vi "Main.vi"(7 "sweep rate, /min":dbl=0.2, 8 "sweep to:":dbl=4.0, 9 "sweep":T8(radio)=enum."2636a_smub") -> ()   [LabVIEW 2021] (continued)
                          n4492 = property on="Offset_super" class="DigNum (strict)"() -> ("Value"=w5886:dbl)  [unwired: 2 in, 2 out]
                          n4493 = property on="Slope_super" class="DigNum (strict)"() -> ("Value"=w5887:dbl)  [unwired: 2 in, 2 out]
                          n4494 = Multiply(x=w5893, y=w5887) -> (x*y=w5892:dbl)
                          n4495 = Add(x=w5892, y=w5886) -> (x+y=w5889:dbl)
                          n4496 = call "setLevel.vi"("VISA resource name 2"=w5888, "Source"=Source."Voltage", "Channel"=Channel."a", "SourceLevel"=w5889) -> ()  [unwired: 1 in, 3 out]
                        }
                      }
                      n4497 = property on="SuperHyper" class="DigNum (strict)"("Value"=w5874) -> ()  [unwired: 2 in, 2 out]
                    }
                  }
                  frame "time_SuperHyper", Default {
                    # "do not sweep, just time"
                  }
                  frame "iPS_SuperHyper" {
                    # "step magnetic field"
                    n4498 = stacked-sequence {
                      tunnel: w5894 -> [_ _ _ _ w5909 _ _ _ w5921 _ w5924 _]
                      frame #0 {
                        n4499 = property on="SuperHyper_Index" class="DigNum (strict)"() -> ("Value"=w5895:dbl)  [unwired: 2 in, 2 out]
                        n4500 = Equal?(x=w5895, y=0.0) -> (x = y?=w5896:bool)
                        n4501 = case shown="True" w5896 {
                          frame False {
                          }
                          frame True {
                            n4502 = property on="iPS _addr_superhyper" class="VISAName"() -> ("Value"=w5900:refnum<visa-resource-name>)  [unwired: 2 in, 2 out]
                            n4503 = property on="Super_FieldRate\n(T/min)" class="DigNum (strict)"() -> ("Value"=w5899:dbl)  [unwired: 2 in, 2 out]
                            n4504 = call "iPSset.vi"("Field Rate, T/min"=w5899, "iPSSetCtrl"=iPSsetCtrl."Set Target Field Rate", "VISA resource name"=w5900) -> ("VISA resource name out"=w5898:refnum<visa-resource-name>)  [unwired: 5 in, 3 out]
                            n4505 = property on="iPS _addr_superhyper" class="VISAName"("Value"=w5898) -> ()  [unwired: 2 in, 2 out]
                          }
                        }
                      }
                      frame #1 {
                        n4506 = Wait (ms)(milliseconds to wait=u32 500) -> ()  [unwired: 1 out]
                      }
                      frame #2 {
                        n4507 = property on="iPS _addr_superhyper" class="VISAName"() -> ("Value"=w5904:refnum<visa-resource-name>)  [unwired: 2 in, 2 out]
                        n4508 = call "iPSset.vi"("iPSSetCtrl"=iPSsetCtrl."Hold", "VISA resource name"=w5904) -> ("VISA resource name out"=w5903:refnum<visa-resource-name>)  [unwired: 6 in, 3 out]
                        n4509 = property on="iPS _addr_superhyper" class="VISAName"("Value"=w5903) -> ()  [unwired: 2 in, 2 out]
                      }
                      frame #3 {
                        n4510 = Wait (ms)(milliseconds to wait=u32 500) -> ()  [unwired: 1 out]
                      }
                      frame #4 {
                        n4511 = property on="iPS _addr_superhyper" class="VISAName"() -> ("Value"=w5908:refnum<visa-resource-name>)  [unwired: 2 in, 2 out]
                        n4512 = call "iPSset.vi"("Target Field, T"=w5909, "iPSSetCtrl"=iPSsetCtrl."Set Target Field", "VISA resource name"=w5908) -> ("VISA resource name out"=w5907:refnum<visa-resource-name>)  [unwired: 5 in, 3 out]
                        n4513 = property on="iPS _addr_superhyper" class="VISAName"("Value"=w5907) -> ()  [unwired: 2 in, 2 out]
                      }
                      frame #5 {
                        n4514 = Wait (ms)(milliseconds to wait=u32 500) -> ()  [unwired: 1 out]
                      }
                      frame #6 {
                        n4515 = property on="iPS _addr_superhyper" class="VISAName"() -> ("Value"=w5912:refnum<visa-resource-name>)  [unwired: 2 in, 2 out]
                        n4516 = call "iPSset.vi"("iPSSetCtrl"=iPSsetCtrl."Hold", "VISA resource name"=w5912) -> ("VISA resource name out"=w5913:refnum<visa-resource-name>)  [unwired: 6 in, 3 out]
                        n4517 = property on="iPS _addr_superhyper" class="VISAName"("Value"=w5913) -> ()  [unwired: 2 in, 2 out]
                      }
                      frame #7 {
                        n4518 = Wait (ms)(milliseconds to wait=u32 500) -> ()  [unwired: 1 out]
                      }
                      frame #8 {
                        n4519 = Equal To 0?(x=w5921) -> (x = 0?=w5920:bool)
                        n4520 = property on="iPS _addr_superhyper" class="VISAName"() -> ("Value"=w5916:refnum<visa-resource-name>)  [unwired: 2 in, 2 out]
                        n4521 = Select(t=iPSsetCtrl."Go to Zero" ("iPSSetCtrl"), s=w5920, f=iPSsetCtrl."Go to Field" ("iPSSetCtrl")) -> (s? t:f=w5917:T16)
                        n4522 = call "iPSset.vi"("iPSSetCtrl"=w5917, "VISA resource name"=w5916) -> ()  [unwired: 6 in, 4 out]
                      }
                      frame #9 {
                        n4523 = Wait (ms)(milliseconds to wait=u32 500) -> ()  [unwired: 1 out]
                      }
                      frame #10 {
                        n4524 = while {
                          tunnel: w5924 -> [w5955]
                          stop <- w5948 stop-if-true
                          n4525 = property on="iPS _addr_superhyper" class="VISAName"() -> ("Value"=w5951:refnum<visa-resource-name>)  [unwired: 2 in, 2 out]
                          n4526 = call "iPSread.vi"("iPSreadCtrl"=iPSreadCtrl."MagnetField", "VISA resource name"=w5951) -> ("number"=w5949:dbl, "VISA resource name out"=w5950:refnum<visa-resource-name>)  [unwired: 6 in, 2 out]
                          n4527 = property on="Tolerance_super" class="DigNum (strict)"() -> ("Value"=w5947:dbl)  [unwired: 2 in, 2 out]
                          n4528 = Wait (ms)(milliseconds to wait=u32 500) -> ()  [unwired: 1 out]
                          n4529 = Subtract(x=w5949, y=w5955) -> (x-y=w5954:dbl)
                          n4530 = property on="iPS _addr_superhyper" class="VISAName"("Value"=w5950) -> ()  [unwired: 2 in, 2 out]
                          n4531 = Absolute Value(x=w5954) -> (abs(x)=w5953:dbl)
                          n4532 = Less Or Equal?(x=w5953, y=w5947) -> (x <= y?=w5948:bool)
                          n4533 = property on="SuperHyper" class="DigNum (strict)"("Value"=w5949) -> ()  [unwired: 2 in, 2 out]
                          n4534 = property on="at field_super" class="Bool (strict)"("Value"=w5948) -> ()  [unwired: 2 in, 2 out]
                        }
                        n4535 = property on="diagona_super" class="Bool (strict)"() -> ("Value"=w5923:bool)  [unwired: 2 in, 2 out]
                        n4536 = case shown="True" w5923 {
                          tunnel: w5924 -> [_ w5932]
                          frame False {
                          }
                          frame True {
                            n4537 = property on="Channel" class="Enum (strict)"() -> ("Value"=w5925:T3)  [unwired: 2 in, 2 out]
                            n4538 = property on="Offset_super" class="DigNum (strict)"() -> ("Value"=w5928:dbl)  [unwired: 2 in, 2 out]
                            n4539 = property on="2336A_addr_super" class="VISAName"() -> ("Value"=w5926:refnum<visa-resource-name>)  [unwired: 2 in, 2 out]
                            n4540 = property on="Slope_super" class="DigNum (strict)"() -> ("Value"=w5929:dbl)  [unwired: 2 in, 2 out]
                            n4541 = call "SinglePointMeasurement.vi"("Measure"=Measure."Voltage", "Channel"=w5925, "VISA resource name 2"=w5926) -> ("Measuremet"=w5930:dbl)  [unwired: 3 in, 4 out]
                            n4542 = Multiply(x=w5932, y=w5929) -> (x*y=w5936:dbl)
                            n4543 = property on="Super_ministeps" class="DigNum (strict)"() -> ("Value"=w5927:dbl)  [unwired: 2 in, 2 out]
                            n4544 = Add(x=w5936, y=w5928) -> (x+y=w5933:dbl)
                            n4545 = Subtract(x=w5933, y=w5930) -> (x-y=w5934:dbl)
                            n4546 = Divide(x=w5934, y=w5927) -> (x/y=w5935:dbl)
                            n4547 = for {
                              N: w5927 -> [_]
                              tunnel: w5935 -> [w5945]
                              tunnel: w5926 -> [w5942]
                              tunnel: w5930 -> [w5938]
                              i -> [w5940]
                              n4548 = Increment(x=w5940) -> (x+1=w5939:i32)
                              n4549 = Multiply(x=w5945, y=w5939) -> (x*y=w5944:dbl)
                              n4550 = Add(x=w5944, y=w5938) -> (x+y=w5941:dbl)
                              n4551 = property on="Channel 2" class="Enum (strict)"() -> ("Value"=w5937:T3)  [unwired: 2 in, 2 out]
                              n4552 = Wait (ms)(milliseconds to wait=u32 12) -> ()  [unwired: 1 out]
                              n4553 = call "setLevel.vi"("VISA resource name 2"=w5942, "Source"=Source."Voltage", "Channel"=w5937, "SourceLevel"=w5941) -> ()  [unwired: 1 in, 3 out]
                            }
                          }
                        }
                      }
                      frame #11 {
                        n4554 = Wait (ms)(milliseconds to wait=u32 500) -> ()  [unwired: 1 out]
                      }
                    }
                  }
                  frame "iTC_SuperHyper" {
                    # "step temperature"
                    n4555 = stacked-sequence {
                      tunnel: w5958 -> [w5966 w5970 w5976]
                      frame #0 {
                        n4556 = Decrement(x=w5966) -> (x-1=w5963:dbl)
                        n4557 = property on="iTC_addr_super" class="VISAName"() -> ("Value"=w5960:refnum<visa-resource-name>)  [unwired: 2 in, 2 out]
                        n4558 = Less Or Equal To 0?(x=w5963) -> (x <= 0?=w5965:bool)
                        n4559 = Select(t=0.0, s=w5965, f=w5963) -> (s? t:f=w5962:dbl)
                        n4560 = call "iTCset.vi"("Set Point"=w5962, "iTCSetCtrl"=iTCsetCtrl."Set VTI Temp", "VISA resource name"=w5960) -> ("VISA resource name out"=w5959:refnum<visa-resource-name>)  [unwired: 5 in, 3 out]
                        n4561 = Wait (ms)(milliseconds to wait=u32 200) -> ()  [unwired: 1 out]
                        n4562 = property on="iTC_addr_super" class="VISAName"("Value"=w5959) -> ()  [unwired: 2 in, 2 out]
                      }
                      frame #1 {
                        n4563 = property on="iTC_addr_super" class="VISAName"() -> ("Value"=w5969:refnum<visa-resource-name>)  [unwired: 2 in, 2 out]
                        n4564 = Less Or Equal To 0?(x=w5970) -> (x <= 0?=w5974:bool)
                        n4565 = Select(t=0.0, s=w5974, f=w5970) -> (s? t:f=w5972:dbl)
                        n4566 = call "iTCset.vi"("Set Point"=w5972, "iTCSetCtrl"=iTCsetCtrl."Set Sample Temp", "VISA resource name"=w5969) -> ("VISA resource name out"=w5968:refnum<visa-resource-name>)  [unwired: 5 in, 3 out]
                        n4567 = Wait (ms)(milliseconds to wait=u32 200) -> ()  [unwired: 1 out]
                        n4568 = property on="iTC_addr_super" class="VISAName"("Value"=w5968) -> ()  [unwired: 2 in, 2 out]
                      }
                      frame #2 {
                        n4569 = while {
                          tunnel: w5976 -> [w5983]
                          stop <- w5977 stop-if-true
                          n4570 = property on="iTC_addr_super" class="VISAName"() -> ("Value"=w5980:refnum<visa-resource-name>)  [unwired: 2 in, 2 out]
                          n4571 = property on="Tolerance_super" class="DigNum (strict)"() -> ("Value"=w5978:dbl)  [unwired: 2 in, 2 out]
                          n4572 = call "iTCread.vi"("VISA resource name"=w5980, "iTCreadCtrl"=iTCreadCtrl."Sample Temp") -> ("number"=w5979:dbl)  [unwired: 5 in, 3 out]
                          n4573 = Subtract(x=w5979, y=w5983) -> (x-y=w5982:dbl)
                          n4574 = Absolute Value(x=w5982) -> (abs(x)=w5981:dbl)
                          n4575 = property on="SuperHyper" class="DigNum (strict)"("Value"=w5979) -> ()  [unwired: 2 in, 2 out]
                          n4576 = Less?(x=w5981, y=w5978) -> (x < y?=w5977:bool)
                          n4577 = property on="at field_super" class="Bool (strict)"("Value"=w5977) -> ()  [unwired: 2 in, 2 out]
                        }
                      }
                    }
                  }
                }
              }
              frame #1 {
                # "Set current hyper channel and wait expected time"
                n4578 = property on="Current SuperHyper Value" class="DigNum (strict)"() -> ("Value"=w5986:dbl)  [unwired: 2 in, 2 out]
                n4579 = property on="Wait Btwn SuperHyper" class="DigNum (strict)"() -> ("Value"=w5985:i32)  [unwired: 2 in, 2 out]
                n4580 = Multiply(x=w5985, y=1000) -> (x*y=w5987:i32)
                n4581 = property on="SuperHyper" class="DigNum (strict)"("Value"=w5986) -> ()  [unwired: 2 in, 2 out]
                n4582 = Wait (ms)(milliseconds to wait=w5987) -> ()  [unwired: 1 out]
              }
              frame #2 {
                # "Check if need to swap step direction"
                n4583 = property on="SwapHyperDirection" class="Bool (strict)"() -> ("Value"=w5989:bool)  [unwired: 2 in, 2 out]
                n4584 = case shown="True" w5989 {
                  frame False {
                  }
                  frame True {
                    n4585 = stacked-sequence {
                      frame #0 {
                        n4586 = property on="SuperHyper_Index" class="DigNum (strict)"() -> ("Value"=w5990:dbl)  [unwired: 2 in, 2 out]
                        n4587 = Equal To 0?(x=w5990) -> (x = 0?=w5991:bool)
                        n4588 = case shown="False" w5991 {
                          frame False {
                            n4589 = property on="from" class="DigNum (strict)"() -> ("Value"=w5995:dbl)  [unwired: 2 in, 2 out]
                            n4590 = property on="to" class="DigNum (strict)"() -> ("Value"=w5993:dbl)  [unwired: 2 in, 2 out]
                            n4591 = Swap Values(12:w5993, 14:w5995) -> (1:w5992:dbl, 3:w5994:dbl)  [unwired: 1 in]
                            n4592 = property on="from" class="DigNum (strict)"("Value"=w5994) -> ()  [unwired: 2 in, 2 out]
                            n4593 = property on="to" class="DigNum (strict)"("Value"=w5992) -> ()  [unwired: 2 in, 2 out]
                          }
                          frame True {
                          }
                        }
                      }
                      frame #1 {
                        n4594 = property on="Hidden_super_Swap" class="Bool (strict)"() -> ("Value"=w5996:bool)  [unwired: 2 in, 2 out]
                        n4595 = property on="Hidden_super_Swap" class="Bool (strict)"("Val(Sgnl)"=w5996) -> ()  [unwired: 2 in, 2 out]
                      }
                    }
                  }
                }
              }
              frame #3 {
                # "Trigger \"start hyper\" event"
                n4596 = property on="Super Hidden" class="Bool (strict)"() -> ("Value"=w5997:bool)  [unwired: 2 in, 2 out]
                n4597 = property on="Super Hidden" class="Bool (strict)"("Val(Sgnl)"=w5997) -> ()  [unwired: 2 in, 2 out]
              }
            }
            n4598 = property on="Current SuperHyper Value" class="DigNum (strict)"("Value"=w5824) -> ()  [unwired: 2 in, 2 out]
          }
          frame True {
            # "When step values are all finished"
            n4599 = Enqueue Element(queue=w6003, element="Idle") -> ()  [unwired: 2 in, 3 out]
            n4600 = property on="Stop SuperHyper" class="Bool"("DisabledEnum"=T10."Disabled and Grayed Out" ("Disabled")) -> ()  [unwired: 2 in, 2 out]
            n4601 = property on="StartSuperHyper" class="Bool"("DisabledEnum"=T10."Enabled" ("Disabled")) -> ()  [unwired: 2 in, 2 out]
            n4602 = property on="Sweep Direction3" class="Str"("Value"="Finished!" ("Sweep Direction"), "Text.TextColor"=u32 16711680 ("Text.Text Colors:Text Color")) -> ()  [unwired: 2 in, 2 out]
          }
        }
      }
      frame "Quit" {
      }
    }
  }
  n4603 = while {
    tunnel: w3 -> [w6008]
    tunnel: w2 -> [w6006]
    tunnel: w1 -> [w6005]
    stop <- w6007 stop-if-true
    # "This loop is the producer loop."
    n4604 = event shown="[14] \"Stop Mapping\": Value Change" {
      selector: _ -> [_ _ _ _ _ _ _ _ _ _ _ _ _ _ _ _ _ _ _ _ _ _ _ _ _ _ _]
      dyn-events: _ -> [_ _ _ _ _ _ _ _ _ _ _ _ _ _ _ _ _ _ _ _ _ _ _ _ _ _ _]
      timeout: _ -> [_ _ _ _ _ _ _ _ _ _ _ _ _ _ _ _ _ _ _ _ _ _ _ _ _ _ _]
      tunnel: w6008 -> [_ w6010 _ _ _ _ _ w6096 _ _ _ _ _ _ w6427 w6432 w6437 w6440 w6447 w6455 w6460 w6464 w6553 w6607 _ _ _]
      tunnel: [_ _ _ _ _ _ _ "Quit" _ _ _ _ _ _ _ _ _ _ _ _ _ _ _ _ _ _ _] -> w6007
      tunnel: w6006 -> [_ _ _ _ _ _ _ _ _ _ _ _ _ _ _ _ _ _ _ _ _ _ _ _ _ w6665 _]
      tunnel: w6005 -> [_ _ _ _ _ _ _ _ _ _ _ _ _ _ _ _ _ _ _ _ _ _ _ _ _ _ w6690]
      event Timeout {
        n4605 = event-data() -> ()  [unwired: 1 in, 3 out]
      }
      event "Initialize": Value Change {
        n4606 = event-data() -> ()  [unwired: 1 in, 6 out]
        n4607 = Enqueue Element(queue=w6010, element="Idle") -> ()  [unwired: 2 in, 3 out]
      }
      event "Linetrace or Mapping?": Value Change {
        n4608 = event-data() -> ()  [unwired: 1 in, 1 out]
        n4609 = case shown="True" "Linetrace or Mapping?" {
          frame True {
            w6017 = T10."Enabled" ("Disabled")
            w6019 = T10."Disabled and Grayed Out" ("Disabled")
            n4610 = property on="Ramp\n Down" class="Bool"("DisabledEnum"=w6019) -> ()  [unwired: 2 in, 2 out]
            n4611 = property on="sweep" class="RadioBtnsControl (strict)"("DisabledEnum"=w6019) -> ()  [unwired: 2 in, 2 out]
            n4612 = property on="2182A 1 addr" class="DigNum (strict)"("DisabledEnum"=w6019) -> ()  [unwired: 2 in, 2 out]
            n4613 = property on="2182A 2 addr" class="DigNum (strict)"("DisabledEnum"=w6019) -> ()  [unwired: 2 in, 2 out]
            n4614 = property on="2182A 3 addr" class="DigNum (strict)"("DisabledEnum"=w6019) -> ()  [unwired: 2 in, 2 out]
            n4615 = property on="2182A 4 addr" class="DigNum (strict)"("DisabledEnum"=w6019) -> ()  [unwired: 2 in, 2 out]
            n4616 = property on="2400 1 addr" class="DigNum (strict)"("DisabledEnum"=w6019) -> ()  [unwired: 2 in, 2 out]
            n4617 = property on="iPS_addr_sweep" class="VISAName"("DisabledEnum"=w6019) -> ()  [unwired: 2 in, 2 out]
            n4618 = property on="Sweep Down" class="Bool"("DisabledEnum"=w6019) -> ()  [unwired: 2 in, 2 out]
            n4619 = property on="SR830 2 addr" class="DigNum (strict)"("DisabledEnum"=w6019) -> ()  [unwired: 2 in, 2 out]
            n4620 = property on="SR830 3 addr" class="DigNum (strict)"("DisabledEnum"=w6019) -> ()  [unwired: 2 in, 2 out]
            n4621 = property on="2400 2 addr" class="DigNum (strict)"("DisabledEnum"=w6019) -> ()  [unwired: 2 in, 2 out]
            n4622 = property on="2400 3 addr" class="DigNum (strict)"("DisabledEnum"=w6019) -> ()  [unwired: 2 in, 2 out]
            n4623 = property on="2614A addr" class="VISAName"("DisabledEnum"=w6019) -> ()  [unwired: 2 in, 2 out]
            n4624 = property on="SR830 1 addr" class="DigNum (strict)"("DisabledEnum"=w6019) -> ()  [unwired: 2 in, 2 out]
            n4625 = property on="SR830 4 addr" class="DigNum (strict)"("DisabledEnum"=w6019) -> ()  [unwired: 2 in, 2 out]
            n4626 = property on="Ramp \nUp" class="Bool"("DisabledEnum"=w6019) -> ()  [unwired: 2 in, 2 out]
            n4627 = property on="Step and Hyerloop Setups" class="TabCtl (strict)"() -> ("Pages"=w6014:refnum<vi>[])  [unwired: 2 in, 2 out]
            n4628 = property on="Sweep Up" class="Bool"("DisabledEnum"=w6019) -> ()  [unwired: 2 in, 2 out]
            n4629 = property on="Tolerance_Sweep" class="DigNum (strict)"("DisabledEnum"=w6019) -> ()  [unwired: 2 in, 2 out]
            n4630 = property on="Continuous Sweep" class="Bool (strict)"("DisabledEnum"=w6019) -> ()  [unwired: 2 in, 2 out]
            n4631 = Index Array(array=w6014, index=2) -> (element=w6015:refnum<vi>)
            n4632 = property on="Continuous Sweep" class="Bool (strict)"("Value"=FALSE ("Continuous Sweep")) -> ()  [unwired: 2 in, 2 out]
            n4633 = property class="Page"(reference=w6015, "PageVis"=FALSE ("Page Visible")) -> ()  [unwired: 1 in, 2 out]
            n4634 = property on="MappingName" class="Str"("Visible"=TRUE) -> ()  [unwired: 2 in, 2 out]
            n4635 = property on="SuperHyper" class="Bool (strict)"("Value"=FALSE ("SuperHyper")) -> ()  [unwired: 2 in, 2 out]
            n4636 = property on="step" class="RadioBtnsControl (strict)"("DisabledEnum"=w6017) -> ()  [unwired: 2 in, 2 out]
            n4637 = property on="diagonal step" class="Bool (strict)"("DisabledEnum"=w6017) -> ()  [unwired: 2 in, 2 out]
            n4638 = property on="Step Offset" class="DigNum (strict)"("DisabledEnum"=w6017) -> ()  [unwired: 2 in, 2 out]
            n4639 = property on="Step Slope" class="DigNum (strict)"("DisabledEnum"=w6017) -> ()  [unwired: 2 in, 2 out]
            n4640 = property on="FieldRate(T/min)" class="DigNum (strict)"("DisabledEnum"=w6017) -> ()  [unwired: 2 in, 2 out]
            n4641 = property on="iPS _addr_step" class="VISAName"("DisabledEnum"=w6017) -> ()  [unwired: 2 in, 2 out]
            n4642 = property on="wait between sweeps(s)" class="DigNum (strict)"("DisabledEnum"=w6017) -> ()  [unwired: 2 in, 2 out]
            n4643 = property on="2614A_addr_step" class="VISAName"("DisabledEnum"=w6017) -> ()  [unwired: 2 in, 2 out]
            n4644 = property on="Start Mapping" class="Bool"("DisabledEnum"=w6017) -> ()  [unwired: 2 in, 2 out]
            n4645 = property on="2400_1_addr_step" class="DigNum (strict)"("DisabledEnum"=w6017) -> ()  [unwired: 2 in, 2 out]
            n4646 = property on="Tolerance_Step" class="DigNum (strict)"("DisabledEnum"=w6017) -> ()  [unwired: 2 in, 2 out]
            n4647 = property on="Wait Between Step(s)" class="DigNum (strict)"("DisabledEnum"=w6017) -> ()  [unwired: 2 in, 2 out]
            n4648 = property on="2400_2_addr_step" class="DigNum (strict)"("DisabledEnum"=w6017) -> ()  [unwired: 2 in, 2 out]
            n4649 = property on="HyperLoop" class="Bool (strict)"("DisabledEnum"=w6017) -> ()  [unwired: 2 in, 2 out]
          }
          frame False {
            w6026 = T10."Disabled and Grayed Out" ("Disabled")
            w6033 = T10."Enabled" ("Disabled")
            n4650 = property on="Ramp\n Down" class="Bool"("DisabledEnum"=w6033) -> ()  [unwired: 2 in, 2 out]
            n4651 = property on="sweep" class="RadioBtnsControl (strict)"("DisabledEnum"=w6033) -> ()  [unwired: 2 in, 2 out]
            n4652 = property on="2182A 1 addr" class="DigNum (strict)"("DisabledEnum"=w6033) -> ()  [unwired: 2 in, 2 out]
            n4653 = property on="2182A 2 addr" class="DigNum (strict)"("DisabledEnum"=w6033) -> ()  [unwired: 2 in, 2 out]
            n4654 = property on="2182A 3 addr" class="DigNum (strict)"("DisabledEnum"=w6033) -> ()  [unwired: 2 in, 2 out]
            n4655 = property on="2182A 4 addr" class="DigNum (strict)"("DisabledEnum"=w6033) -> ()  [unwired: 2 in, 2 out]
            n4656 = property on="2400 1 addr" class="DigNum (strict)"("DisabledEnum"=w6033) -> ()  [unwired: 2 in, 2 out]
            n4657 = property on="iPS_addr_sweep" class="VISAName"("DisabledEnum"=w6033) -> ()  [unwired: 2 in, 2 out]
            n4658 = property on="Sweep Down" class="Bool"("DisabledEnum"=w6033) -> ()  [unwired: 2 in, 2 out]
            n4659 = property on="SR830 2 addr" class="DigNum (strict)"("DisabledEnum"=w6033) -> ()  [unwired: 2 in, 2 out]
            n4660 = property on="SR830 3 addr" class="DigNum (strict)"("DisabledEnum"=w6033) -> ()  [unwired: 2 in, 2 out]
            n4661 = property on="2400 2 addr" class="DigNum (strict)"("DisabledEnum"=w6033) -> ()  [unwired: 2 in, 2 out]
            n4662 = property on="2400 3 addr" class="DigNum (strict)"("DisabledEnum"=w6033) -> ()  [unwired: 2 in, 2 out]
            n4663 = property on="2614A addr" class="VISAName"("DisabledEnum"=w6033) -> ()  [unwired: 2 in, 2 out]
            n4664 = property on="SR830 1 addr" class="DigNum (strict)"("DisabledEnum"=w6033) -> ()  [unwired: 2 in, 2 out]
            n4665 = property on="SR830 4 addr" class="DigNum (strict)"("DisabledEnum"=w6033) -> ()  [unwired: 2 in, 2 out]
            n4666 = property on="Ramp \nUp" class="Bool"("DisabledEnum"=w6033) -> ()  [unwired: 2 in, 2 out]
            n4667 = property on="Sweep Up" class="Bool"("DisabledEnum"=w6033) -> ()  [unwired: 2 in, 2 out]
            n4668 = property on="Step and Hyerloop Setups" class="TabCtl (strict)"() -> ("Pages"=w6021:refnum<vi>[])  [unwired: 2 in, 2 out]
            n4669 = property on="Tolerance_Sweep" class="DigNum (strict)"("DisabledEnum"=w6033) -> ()  [unwired: 2 in, 2 out]
            n4670 = property on="Continuous Sweep" class="Bool (strict)"("DisabledEnum"=w6033) -> ()  [unwired: 2 in, 2 out]
            n4671 = property on="Step and Hyerloop Setups" class="TabCtl (strict)"() -> ("Pages"=w6031:refnum<vi>[])  [unwired: 2 in, 2 out]
            n4672 = Index Array(array=w6021, index=2) -> (element=w6022:refnum<vi>)
            n4673 = property on="MappingName" class="Str"("Visible"=FALSE) -> ()  [unwired: 2 in, 2 out]
            n4674 = property on="SuperHyper" class="Bool (strict)"("Value"=FALSE ("SuperHyper")) -> ()  [unwired: 2 in, 2 out]
            n4675 = Index Array(array=w6031, index=1) -> (element=w6030:refnum<vi>)
            n4676 = property class="Page"(reference=w6022, "PageVis"=FALSE ("Page Visible")) -> ()  [unwired: 1 in, 2 out]
            n4677 = property on="HyperLoop" class="Bool (strict)"("Value"=FALSE ("HyperLoop")) -> ()  [unwired: 2 in, 2 out]
            n4678 = property class="Page"(reference=w6030, "PageVis"=FALSE ("Page Visible")) -> ()  [unwired: 1 in, 2 out]
            n4679 = property on="step" class="RadioBtnsControl (strict)"("DisabledEnum"=w6026) -> ()  [unwired: 2 in, 2 out]
            n4680 = property on="diagonal step" class="Bool (strict)"("DisabledEnum"=w6026) -> ()  [unwired: 2 in, 2 out]
            n4681 = property on="Step Offset" class="DigNum (strict)"("DisabledEnum"=w6026) -> ()  [unwired: 2 in, 2 out]
            n4682 = property on="Step Slope" class="DigNum (strict)"("DisabledEnum"=w6026) -> ()  [unwired: 2 in, 2 out]
            n4683 = property on="iPS _addr_step" class="VISAName"("DisabledEnum"=w6026) -> ()  [unwired: 2 in, 2 out]
            n4684 = property on="wait between sweeps(s)" class="DigNum (strict)"("DisabledEnum"=w6026) -> ()  [unwired: 2 in, 2 out]
            n4685 = property on="2614A_addr_step" class="VISAName"("DisabledEnum"=w6026) -> ()  [unwired: 2 in, 2 out]
            n4686 = property on="Start Mapping" class="Bool"("DisabledEnum"=w6026) -> ()  [unwired: 2 in, 2 out]
            n4687 = property on="2400_1_addr_step" class="DigNum (strict)"("DisabledEnum"=w6026) -> ()  [unwired: 2 in, 2 out]
            n4688 = property on="Wait Between Step(s)" class="DigNum (strict)"("DisabledEnum"=w6026) -> ()  [unwired: 2 in, 2 out]
            n4689 = property on="2400_2_addr_step" class="DigNum (strict)"("DisabledEnum"=w6026) -> ()  [unwired: 2 in, 2 out]
            n4690 = property on="FieldRate(T/min)" class="DigNum (strict)"("DisabledEnum"=w6026) -> ()  [unwired: 2 in, 2 out]
            n4691 = property on="Tolerance_Step" class="DigNum (strict)"("DisabledEnum"=w6026) -> ()  [unwired: 2 in, 2 out]
            n4692 = property on="HyperLoop" class="Bool (strict)"("DisabledEnum"=w6026) -> ()  [unwired: 2 in, 2 out]
          }
        }
      }
      event "Change Sweep Range": Value Change {
        n4693 = event-data() -> ()  [unwired: 1 in, 6 out]
        n4694 = property on="Change Sweep Range" class="Bool (strict)"() -> ("Value"=w6034:bool)  [unwired: 2 in, 2 out]
        n4695 = case shown="False" w6034 {
          frame False {
            w6035 = FALSE ("Visible")
            n4696 = property on="UpLimitValue" class="DigNum (strict)"("Visible"=w6035) -> ()  [unwired: 2 in, 2 out]
            n4697 = property on="DownLimitValue" class="DigNum (strict)"("Visible"=w6035) -> ()  [unwired: 2 in, 2 out]
            n4698 = property on="Generate" class="Bool"("Visible"=w6035) -> ()  [unwired: 2 in, 2 out]
            n4699 = property on="Offset_Up" class="DigNum (strict)"("Visible"=w6035) -> ()  [unwired: 2 in, 2 out]
            n4700 = property on="Down          Up" class="Tbl (strict)"("Visible"=w6035) -> ()  [unwired: 2 in, 2 out]
            n4701 = property on="Slope" class="DigNum (strict)"("Visible"=w6035) -> ()  [unwired: 2 in, 2 out]
            n4702 = property on="Offset_Down" class="DigNum (strict)"("Visible"=w6035) -> ()  [unwired: 2 in, 2 out]
          }
          frame True {
            w6036 = TRUE ("Visible")
            n4703 = property on="UpLimitValue" class="DigNum (strict)"("Visible"=w6036) -> ()  [unwired: 2 in, 2 out]
            n4704 = property on="Generate" class="Bool"("Visible"=w6036) -> ()  [unwired: 2 in, 2 out]
            n4705 = property on="DownLimitValue" class="DigNum (strict)"("Visible"=w6036) -> ()  [unwired: 2 in, 2 out]
            n4706 = property on="Offset_Up" class="DigNum (strict)"("Visible"=w6036) -> ()  [unwired: 2 in, 2 out]
            n4707 = property on="Down          Up" class="Tbl (strict)"("Visible"=w6036) -> ()  [unwired: 2 in, 2 out]
            n4708 = property on="Slope" class="DigNum (strict)"("Visible"=w6036) -> ()  [unwired: 2 in, 2 out]
            n4709 = property on="Offset_Down" class="DigNum (strict)"("Visible"=w6036) -> ()  [unwired: 2 in, 2 out]
          }
        }
      }
      event "Generate": Value Change {
        n4710 = event-data() -> ()  [unwired: 1 in, 6 out]
        n4711 = stacked-sequence {
          frame #0 {
            # "Initialize the background colours of cells"
            n4712 = property on="Down          Up" class="Tbl (strict)"("Active Cell"=cluster{"Row":i32, "Column":i32} {"Row"=-2, "Column"=-2}, "Cell BG Color"=u32 16448250 ("Active Cell:Cell Background Color")) -> ()  [unwired: 2 in, 2 out]
          }
          frame #1 {
            # "Fill the tables"
            n4713 = property on="Step values" class="Tbl (strict)"() -> ("Value"=w6046:string[][])  [unwired: 2 in, 2 out]
            n4714 = Index Array(array=w6046, index (col)=0 ("index (row)")) -> (element=w6043:string[])  [unwired: 1 in]
            n4715 = Array Size(array=w6043) -> (size(s)=w6045:i32)
            n4716 = for {
              N: w6045 -> [_]
              tunnel: [w6063] -> w6042 mode=indexing
              tunnel: [w6062] -> w6041 mode=indexing
              i -> [w6059]
              n4717 = property on="Step values" class="Tbl (strict)"() -> ("Value"=w6061:string[][])  [unwired: 2 in, 2 out]
              n4718 = property on="Slope" class="DigNum (strict)"() -> ("Value"=w6065:dbl)  [unwired: 2 in, 2 out]
              n4719 = Index Array(array=w6061, index (row)=w6059, index (col)=0 ("disabled index (col)")) -> (element=w6058:string)
              n4720 = Fract/Exp String To Number(string=w6058) -> (number=w6057:dbl)  [unwired: 3 in, 1 out]
              n4721 = property on="Offset_Up" class="DigNum (strict)"() -> ("Value"=w6064:dbl)  [unwired: 2 in, 2 out]
              n4722 = Multiply(x=w6057, y=w6065) -> (x*y=w6054:dbl)
              n4723 = property on="Offset_Down" class="DigNum (strict)"() -> ("Value"=w6055:dbl)  [unwired: 2 in, 2 out]
              n4724 = property on="UpLimitValue" class="DigNum (strict)"() -> ("Value"=w6048:dbl)  [unwired: 2 in, 2 out]
              n4725 = Add(x=w6054, y=w6064) -> (x+y=w6049:dbl)
              n4726 = Add(x=w6055, y=w6054) -> (x+y=w6053:dbl)
              n4727 = property on="DownLimitValue" class="DigNum (strict)"() -> ("Value"=w6052:dbl)  [unwired: 2 in, 2 out]
              n4728 = Less?(x=w6049, y=w6048) -> (x < y?=w6050:bool)
              n4729 = Greater?(x=w6053, y=w6052) -> (0:w6056:bool)
              n4730 = Select(t=w6049, s=w6050, f=w6048) -> (s? t:f=w6047:dbl)
              n4731 = Select(t=w6053, s=w6056, f=w6052) -> (s? t:f=w6051:dbl)
              n4732 = Number To Fractional String(number=w6051) -> (F-format string=w6063:string)  [unwired: 3 in]
              n4733 = Number To Fractional String(number=w6047) -> (F-format string=w6062:string)  [unwired: 3 in]
            }
            n4734 = Build Array(w6042, w6041) -> (w6040:string[][])
            n4735 = Transpose 2D Array(2D array=w6040) -> (transposed array=w6039:string[][])
            n4736 = property on="Down          Up" class="Tbl (strict)"("Value"=w6039) -> ()  [unwired: 2 in, 2 out]
          }
        }
      }
      event "HyperLoop": Value Change {
        n4737 = event-data() -> ()  [unwired: 1 in, 6 out]
        n4738 = property on="HyperLoop" class="Bool (strict)"() -> ("Value"=w6066:bool)  [unwired: 2 in, 2 out]
        n4739 = case shown="True" w6066 {
          frame False {
            n4740 = property on="Step and Hyerloop Setups" class="TabCtl (strict)"() -> ("Pages"=w6072:refnum<vi>[])  [unwired: 2 in, 2 out]
            n4741 = Index Array(array=w6072, index=2) -> (element=w6071:refnum<vi>)
            n4742 = property on="SuperHyper" class="Bool (strict)"("Value"=FALSE ("SuperHyper")) -> ()  [unwired: 2 in, 2 out]
            n4743 = property on="HyperLoop" class="Bool (strict)"("Value"=FALSE ("HyperLoop")) -> ()  [unwired: 2 in, 2 out]
            n4744 = property class="Page"(reference=w6071, "PageVis"=FALSE ("Page Visible")) -> ()  [unwired: 1 in, 2 out]
            n4745 = property on="Step and Hyerloop Setups" class="TabCtl (strict)"() -> ("Pages"=w6077:refnum<vi>[])  [unwired: 2 in, 2 out]
            n4746 = Index Array(array=w6077, index=1) -> (element=w6076:refnum<vi>)
            n4747 = property on="Start Mapping" class="Bool"("DisabledEnum"=T10."Enabled" ("Disabled")) -> ()  [unwired: 2 in, 2 out]
            n4748 = property class="Page"(reference=w6076, "PageVis"=FALSE ("Page Visible")) -> ()  [unwired: 1 in, 2 out]
          }
          frame True {
            n4749 = property on="Step and Hyerloop Setups" class="TabCtl (strict)"() -> ("Pages"=w6083:refnum<vi>[])  [unwired: 2 in, 2 out]
            n4750 = Index Array(array=w6083, index=1) -> (element=w6081:refnum<vi>)
            n4751 = property on="Start Mapping" class="Bool"("DisabledEnum"=T10."Disabled and Grayed Out" ("Disabled")) -> ()  [unwired: 2 in, 2 out]
            n4752 = property class="Page"(reference=w6081, "PageVis"=TRUE ("Page Visible")) -> ()  [unwired: 1 in, 2 out]
            n4753 = property on="SuperHyper" class="Bool (strict)"("Value"=FALSE ("SuperHyper")) -> ()  [unwired: 2 in, 2 out]
          }
        }
      }
      event "SuperHyper": Value Change {
        n4754 = event-data() -> ()  [unwired: 1 in, 6 out]
        n4755 = property on="SuperHyper" class="Bool (strict)"() -> ("Value"=w6084:bool)  [unwired: 2 in, 2 out]
        n4756 = case shown="False" w6084 {
          frame False {
            n4757 = property on="Step and Hyerloop Setups" class="TabCtl (strict)"() -> ("Pages"=w6089:refnum<vi>[])  [unwired: 2 in, 2 out]
            n4758 = Index Array(array=w6089, index=2) -> (element=w6088:refnum<vi>)
            n4759 = property on="Start HyperLoop" class="Bool"("DisabledEnum"=T10."Enabled" ("Disabled")) -> ()  [unwired: 2 in, 2 out]
            n4760 = property class="Page"(reference=w6088, "PageVis"=FALSE ("Page Visible")) -> ()  [unwired: 1 in, 2 out]
          }
          frame True {
            n4761 = property on="Step  Setups" class="TabCtl (strict)"() -> ("Pages"=w6094:refnum<vi>[])  [unwired: 2 in, 2 out]
            n4762 = Index Array(array=w6094, index=2) -> (element=w6092:refnum<vi>)
            n4763 = property class="Page"(reference=w6092, "PageVis"=TRUE ("Page Visible")) -> ()  [unwired: 1 in, 2 out]
            n4764 = property on="Start HyperLoop" class="Bool"("DisabledEnum"=T10."Disabled and Grayed Out" ("Disabled")) -> ()  [unwired: 2 in, 2 out]
          }
        }
      }
      event "Quit": Value Change {
        n4765 = event-data() -> ()  [unwired: 1 in, 6 out]
        n4766 = Flush Queue(queue=w6096) -> (queue out=w6095:refnum<queue>)  [unwired: 1 in, 2 out]
        n4767 = Enqueue Element(queue=w6095, element="Quit") -> ()  [unwired: 2 in, 3 out]
      }
      event "Populate step table?": Value Change {
        n4768 = event-data() -> ()  [unwired: 1 in, 6 out]
        n4769 = stacked-sequence {
          frame #0 {
            # "Initialize the background colours of cells"
            n4770 = property on="Step values" class="Tbl (strict)"("Active Cell"=cluster{"Row":i32, "Column":i32} {"Row"=-2, "Column"=-2}, "Cell BG Color"=u32 16448250 ("Active Cell:Cell Background Color")) -> ()  [unwired: 2 in, 2 out]
          }
          frame #1 {
            # "Fill the tables"
            n4771 = property on="to" class="DigNum (strict)"() -> ("Value"=w6102:dbl)  [unwired: 2 in, 2 out]
            n4772 = property on="step" class="DigNum (strict)"() -> ("Value"=w6101:dbl)  [unwired: 2 in, 2 out]
            n4773 = property on="from" class="DigNum (strict)"() -> ("Value"=w6103:dbl)  [unwired: 2 in, 2 out]
            n4774 = Subtract(x=w6103, y=w6102) -> (x-y=w6110:dbl)
            n4775 = Divide(x=w6110, y=w6101) -> (x/y=w6109:dbl)
            n4776 = Sign(1:w6110) -> (0:w6113:dbl)
            n4777 = Absolute Value(x=w6109) -> (abs(x)=w6108:dbl)
            n4778 = Negate(x=w6113) -> (-x=w6105:dbl)
            n4779 = Round Toward -Infinity(1:w6108) -> (0:w6107:dbl)
            n4780 = Increment(x=w6107) -> (x+1=w6106:dbl)
            n4781 = for {
              N: w6106 -> [_]
              tunnel: w6103 -> [w6119]
              tunnel: w6105 -> [w6120]
              tunnel: w6101 -> [w6122]
              tunnel: [w6116] -> w6111 mode=indexing
              i -> [w6114]
              n4782 = Multiply(x=w6122, y=w6114) -> (x*y=w6121:dbl)
              n4783 = Multiply(x=w6120, y=w6121) -> (x*y=w6118:dbl)
              n4784 = Add(x=w6119, y=w6118) -> (x+y=w6117:dbl)
              n4785 = Number To Fractional String(number=w6117, precision (6)=i16 6) -> (F-format string=w6116:string)  [unwired: 2 in]
            }
            n4786 = Build Array(w6111) -> (w6112:string[][])
            n4787 = Transpose 2D Array(2D array=w6112) -> (transposed array=w6104:string[][])
            n4788 = property on="Step values" class="Tbl (strict)"("Value"=w6104) -> ()  [unwired: 2 in, 2 out]
          }
          frame #2 {
            # "Calculate the measurement time and estimate the finished time"
            n4789 = property on="upper limit" class="DigNum (strict)"() -> ("Value"=w6154:dbl)  [unwired: 2 in, 2 out]
            n4790 = property on="lower limit" class="DigNum (strict)"() -> ("Value"=w6155:dbl)  [unwired: 2 in, 2 out]
            n4791 = Subtract(x=w6155, y=w6154) -> (x-y=w6153:dbl)
            n4792 = property on="Down Rate" class="DigNum (strict)"() -> ("Value"=w6150:dbl)  [unwired: 2 in, 2 out]
            n4793 = property on="Up Rate" class="DigNum (strict)"() -> ("Value"=w6152:dbl)  [unwired: 2 in, 2 out]
            n4794 = Absolute Value(x=w6153) -> (abs(x)=w6151:dbl)
            n4795 = property on="step" class="RadioBtnsControl (strict)"() -> ("Value"=w6130:T5)  [unwired: 2 in, 2 out]
            n4796 = Divide(x=w6151, y=w6152) -> (x/y=w6149:dbl)
            n4797 = Divide(x=w6151, y=w6150) -> (x/y=w6148:dbl)
            n4798 = case shown="\"iPS_step\"" w6130 {
              tunnel: [w6156 0.0] -> w6126
              frame "iPS_step" {
                n4799 = property on="step" class="DigNum (strict)"() -> ("Value"=w6160:dbl)  [unwired: 2 in, 2 out]
                n4800 = property on="FieldRate(T/min)" class="DigNum (strict)"() -> ("Value"=w6159:dbl)  [unwired: 2 in, 2 out]
                n4801 = Divide(x=w6160, y=w6159) -> (x/y=w6158:dbl)
                n4802 = Multiply(x=w6158, y=60.0) -> (x*y=w6156:dbl)
              }
              frame "V2400_1_Step".."iTC_step", Default {
              }
            }
            n4803 = property on="Wait Between Step(s)" class="DigNum (strict)"() -> ("Value"=w6145:i32)  [unwired: 2 in, 2 out]
            n4804 = Add(x=w6149, y=w6148) -> (x+y=w6147:dbl)
            n4805 = Multiply(x=w6147, y=60.0) -> (x*y=w6146:dbl)
            n4806 = property on="Step values" class="Tbl (strict)"() -> ("Value"=w6140:string[][])  [unwired: 2 in, 2 out]
            n4807 = property on="wait between sweeps(s)" class="DigNum (strict)"() -> ("Value"=w6143:u32)  [unwired: 2 in, 2 out]
            n4808 = Add(x=w6146, y=w6145) -> (x+y=w6144:dbl)
            n4809 = Array Size(array=w6140) -> (size(s)=w6139:i32[])
            n4810 = Index Array(array=w6139, index=0) -> (element=w6125:i32)
            n4811 = Add(x=w6144, y=w6143) -> (x+y=w6129:dbl)
            n4812 = Multiply(x=w6125, y=w6129) -> (x*y=w6127:dbl)
            n4813 = Decrement(x=w6125) -> (x-1=w6124:i32)
            n4814 = Multiply(x=w6124, y=w6126) -> (x*y=w6123:dbl)
            n4815 = Add(x=w6127, y=w6123) -> (x+y=w6128:dbl)
            n4816 = Get Date/Time In Seconds() -> (seconds since 1Jan1904=w6142:timestamp)
            n4817 = Add(x=w6128, y=w6142) -> (x+y=w6138:timestamp)
            n4818 = Quotient & Remainder(x=w6128, y=3600.0) -> (x-y*floor(x/y)=w6141:dbl, floor(x/y)=w6137:dbl)
            n4819 = Quotient & Remainder(x=w6141, y=60.0) -> (x-y*floor(x/y)=w6135:dbl, floor(x/y)=w6136:dbl)
            n4820 = property on="SS:" class="DigNum (strict)"("Value"=w6135) -> ()  [unwired: 2 in, 2 out]
            n4821 = property on="MM:" class="DigNum (strict)"("Value"=w6136) -> ()  [unwired: 2 in, 2 out]
            n4822 = property on="HH:" class="DigNum (strict)"("Value"=w6137) -> ()  [unwired: 2 in, 2 out]
            n4823 = property on="Finish Time" class="AbsTime (strict)"("Value"=w6138) -> ()  [unwired: 2 in, 2 out]
          }
        }
      }
      event "Hidden_HyperLoop_Swap": Value Change {
        n4824 = event-data() -> ()  [unwired: 1 in, 6 out]
        n4825 = stacked-sequence {
          frame #0 {
            # "Initialize the background colours of cells"
            n4826 = property on="Step values" class="Tbl (strict)"("Active Cell"=cluster{"Row":i32, "Column":i32} {"Row"=-2, "Column"=-2}, "Cell BG Color"=u32 16448250 ("Active Cell:Cell Background Color")) -> ()  [unwired: 2 in, 2 out]
          }
          frame #1 {
            # "Fill the tables"
            n4827 = property on="Step values" class="Tbl (strict)"() -> ("Value"=w6169:string[][])  [unwired: 2 in, 2 out]
            n4828 = Index Array(array=w6169, index (col)=0 ("disabled index (col)")) -> (element=w6167:string[])  [unwired: 1 in]
            n4829 = Reverse 1D Array(array=w6167) -> (reversed array=w6166:string[])
            n4830 = Build Array(w6166) -> (w6165:string[][])
            n4831 = Transpose 2D Array(2D array=w6165) -> (transposed array=w6164:string[][])
            n4832 = property on="Step values" class="Tbl (strict)"("Value"=w6164) -> ()  [unwired: 2 in, 2 out]
          }
          frame #2 {
            # "Calculate the measurement time and estimate the finished time"
            n4833 = property on="upper limit" class="DigNum (strict)"() -> ("Value"=w6201:dbl)  [unwired: 2 in, 2 out]
            n4834 = property on="lower limit" class="DigNum (strict)"() -> ("Value"=w6202:dbl)  [unwired: 2 in, 2 out]
            n4835 = Subtract(x=w6202, y=w6201) -> (x-y=w6200:dbl)
            n4836 = property on="Down Rate" class="DigNum (strict)"() -> ("Value"=w6197:dbl)  [unwired: 2 in, 2 out]
            n4837 = property on="Up Rate" class="DigNum (strict)"() -> ("Value"=w6199:dbl)  [unwired: 2 in, 2 out]
            n4838 = Absolute Value(x=w6200) -> (abs(x)=w6198:dbl)
            n4839 = property on="step" class="RadioBtnsControl (strict)"() -> ("Value"=w6177:T5)  [unwired: 2 in, 2 out]
            n4840 = Divide(x=w6198, y=w6199) -> (x/y=w6196:dbl)
            n4841 = Divide(x=w6198, y=w6197) -> (x/y=w6195:dbl)
            n4842 = case shown="\"iPS_step\"" w6177 {
              tunnel: [w6203 0.0] -> w6173
              frame "iPS_step" {
                n4843 = property on="step" class="DigNum (strict)"() -> ("Value"=w6207:dbl)  [unwired: 2 in, 2 out]
                n4844 = property on="FieldRate(T/min)" class="DigNum (strict)"() -> ("Value"=w6206:dbl)  [unwired: 2 in, 2 out]
                n4845 = Divide(x=w6207, y=w6206) -> (x/y=w6205:dbl)
                n4846 = Multiply(x=w6205, y=60.0) -> (x*y=w6203:dbl)
              }
              frame "V2400_1_Step".."iTC_step", Default {
              }
            }
            n4847 = property on="Wait Between Step(s)" class="DigNum (strict)"() -> ("Value"=w6192:i32)  [unwired: 2 in, 2 out]
            n4848 = Add(x=w6196, y=w6195) -> (x+y=w6194:dbl)
            n4849 = Multiply(x=w6194, y=60.0) -> (x*y=w6193:dbl)
            n4850 = property on="Step values" class="Tbl (strict)"() -> ("Value"=w6187:string[][])  [unwired: 2 in, 2 out]
            n4851 = property on="wait between sweeps(s)" class="DigNum (strict)"() -> ("Value"=w6190:u32)  [unwired: 2 in, 2 out]
            n4852 = Add(x=w6193, y=w6192) -> (x+y=w6191:dbl)
            n4853 = Array Size(array=w6187) -> (size(s)=w6186:i32[])
            n4854 = Index Array(array=w6186, index=0) -> (element=w6172:i32)
            n4855 = Add(x=w6191, y=w6190) -> (x+y=w6176:dbl)
            n4856 = Multiply(x=w6172, y=w6176) -> (x*y=w6174:dbl)
            n4857 = Decrement(x=w6172) -> (x-1=w6171:i32)
            n4858 = Multiply(x=w6171, y=w6173) -> (x*y=w6170:dbl)
            n4859 = Add(x=w6174, y=w6170) -> (x+y=w6175:dbl)
            n4860 = Get Date/Time In Seconds() -> (seconds since 1Jan1904=w6189:timestamp)
            n4861 = Add(x=w6175, y=w6189) -> (x+y=w6185:timestamp)
            n4862 = Quotient & Remainder(x=w6175, y=3600.0) -> (x-y*floor(x/y)=w6188:dbl, floor(x/y)=w6184:dbl)
            n4863 = Quotient & Remainder(x=w6188, y=60.0) -> (x-y*floor(x/y)=w6182:dbl, floor(x/y)=w6183:dbl)
            n4864 = property on="SS:" class="DigNum (strict)"("Value"=w6182) -> ()  [unwired: 2 in, 2 out]
            n4865 = property on="MM:" class="DigNum (strict)"("Value"=w6183) -> ()  [unwired: 2 in, 2 out]
            n4866 = property on="HH:" class="DigNum (strict)"("Value"=w6184) -> ()  [unwired: 2 in, 2 out]
            n4867 = property on="Finish Time" class="AbsTime (strict)"("Value"=w6185) -> ()  [unwired: 2 in, 2 out]
          }
        }
      }
      event "Populate HyperLoop table?": Value Change {
        n4868 = event-data() -> ()  [unwired: 1 in, 6 out]
        n4869 = stacked-sequence {
          frame #0 {
            n4870 = property on="HyperLoop Steps" class="Tbl (strict)"("Active Cell"=cluster{"Row":i32, "Column":i32} {"Row"=-2, "Column"=-2}, "Cell BG Color"=u32 16448250 ("Active Cell:Cell Background Color")) -> ()  [unwired: 2 in, 2 out]
          }
          frame #1 {
            n4871 = property on="to" class="DigNum (strict)"() -> ("Value"=w6213:dbl)  [unwired: 2 in, 2 out]
            n4872 = property on="step" class="DigNum (strict)"() -> ("Value"=w6212:dbl)  [unwired: 2 in, 2 out]
            n4873 = property on="from" class="DigNum (strict)"() -> ("Value"=w6214:dbl)  [unwired: 2 in, 2 out]
            n4874 = Subtract(x=w6214, y=w6213) -> (x-y=w6220:dbl)
            n4875 = Divide(x=w6220, y=w6212) -> (x/y=w6219:dbl)
            n4876 = Sign(1:w6220) -> (0:w6223:dbl)
            n4877 = Absolute Value(x=w6219) -> (abs(x)=w6218:dbl)
            n4878 = Negate(x=w6223) -> (-x=w6215:dbl)
            n4879 = Round Toward -Infinity(1:w6218) -> (0:w6217:dbl)
            n4880 = Increment(x=w6217) -> (x+1=w6216:dbl)
            n4881 = for {
              N: w6216 -> [_]
              tunnel: w6214 -> [w6229]
              tunnel: w6215 -> [w6230]
              tunnel: w6212 -> [w6232]
              tunnel: [w6226] -> w6221 mode=indexing
              i -> [w6224]
              n4882 = Multiply(x=w6232, y=w6224) -> (x*y=w6231:dbl)
              n4883 = Multiply(x=w6230, y=w6231) -> (x*y=w6228:dbl)
              n4884 = Add(x=w6229, y=w6228) -> (x+y=w6227:dbl)
              n4885 = Number To Fractional String(number=w6227, precision (6)=i16 6) -> (F-format string=w6226:string)  [unwired: 2 in]
            }
            n4886 = Build Array(w6221) -> (w6222:string[][])
            n4887 = Transpose 2D Array(2D array=w6222) -> (transposed array=w6211:string[][])
            n4888 = property on="HyperLoop Steps" class="Tbl (strict)"("Value"=w6211) -> ()  [unwired: 2 in, 2 out]
          }
          frame #2 {
            n4889 = property on="upper limit" class="DigNum (strict)"() -> ("Value"=w6267:dbl)  [unwired: 2 in, 2 out]
            n4890 = property on="lower limit" class="DigNum (strict)"() -> ("Value"=w6268:dbl)  [unwired: 2 in, 2 out]
            n4891 = Subtract(x=w6268, y=w6267) -> (x-y=w6266:dbl)
            n4892 = property on="Down Rate" class="DigNum (strict)"() -> ("Value"=w6263:dbl)  [unwired: 2 in, 2 out]
            n4893 = property on="Up Rate" class="DigNum (strict)"() -> ("Value"=w6265:dbl)  [unwired: 2 in, 2 out]
            n4894 = Absolute Value(x=w6266) -> (abs(x)=w6264:dbl)
            n4895 = property on="step" class="RadioBtnsControl (strict)"() -> ("Value"=w6244:T5)  [unwired: 2 in, 2 out]
            n4896 = Divide(x=w6264, y=w6265) -> (x/y=w6262:dbl)
            n4897 = Divide(x=w6264, y=w6263) -> (x/y=w6261:dbl)
            n4898 = case shown="\"V2400_1_Step\"..\"iTC_step\", Default" w6244 {
              tunnel: [w6269 0.0] -> w6243
              frame "iPS_step" {
                n4899 = property on="step" class="DigNum (strict)"() -> ("Value"=w6273:dbl)  [unwired: 2 in, 2 out]
                n4900 = property on="FieldRate(T/min)" class="DigNum (strict)"() -> ("Value"=w6272:dbl)  [unwired: 2 in, 2 out]
                n4901 = Divide(x=w6273, y=w6272) -> (x/y=w6271:dbl)
                n4902 = Multiply(x=w6271, y=60.0) -> (x*y=w6269:dbl)
              }
              frame "V2400_1_Step".."iTC_step", Default {
              }
            }
            n4903 = property on="Wait Between Step(s)" class="DigNum (strict)"() -> ("Value"=w6258:i32)  [unwired: 2 in, 2 out]
            n4904 = Add(x=w6262, y=w6261) -> (x+y=w6260:dbl)
            n4905 = Multiply(x=w6260, y=60.0) -> (x*y=w6259:dbl)
            n4906 = property on="HyperLoop Steps" class="Tbl (strict)"() -> ("Value"=w6239:string[][])  [unwired: 2 in, 2 out]
            n4907 = property on="wait between sweeps(s)" class="DigNum (strict)"() -> ("Value"=w6256:u32)  [unwired: 2 in, 2 out]
            n4908 = Add(x=w6259, y=w6258) -> (x+y=w6257:dbl)
            n4909 = property on="Step values" class="Tbl (strict)"() -> ("Value"=w6253:string[][])  [unwired: 2 in, 2 out]
            n4910 = Array Size(array=w6239) -> (size(s)=w6241:i32[])
            n4911 = Array Size(array=w6253) -> (size(s)=w6252:i32[])
            n4912 = Add(x=w6257, y=w6256) -> (x+y=w6246:dbl)
            n4913 = Index Array(array=w6241, index=0) -> (element=w6242:i32)
            n4914 = Index Array(array=w6252, index=0) -> (element=w6251:i32)
            n4915 = Add(x=w6246, y=w6243) -> (x+y=w6245:dbl)
            n4916 = Multiply(x=w6251, y=w6245) -> (x*y=w6238:dbl)
            n4917 = Multiply(x=w6242, y=w6238) -> (x*y=w6237:dbl)
            n4918 = Get Date/Time In Seconds() -> (seconds since 1Jan1904=w6255:timestamp)
            n4919 = Add(x=w6237, y=w6255) -> (x+y=w6233:timestamp)
            n4920 = Quotient & Remainder(x=w6237, y=3600.0) -> (x-y*floor(x/y)=w6254:dbl, floor(x/y)=w6234:dbl)
            n4921 = Quotient & Remainder(x=w6254, y=60.0) -> (x-y*floor(x/y)=w6236:dbl, floor(x/y)=w6235:dbl)
            n4922 = property on="Finish Time 2" class="AbsTime (strict)"("Value"=w6233) -> ()  [unwired: 2 in, 2 out]
            n4923 = property on="HH:" class="DigNum (strict)"("Value"=w6234) -> ()  [unwired: 2 in, 2 out]
            n4924 = property on="MM:" class="DigNum (strict)"("Value"=w6235) -> ()  [unwired: 2 in, 2 out]
            n4925 = property on="SS:" class="DigNum (strict)"("Value"=w6236) -> ()  [unwired: 2 in, 2 out]
          }
        }
      }
      event "Populate SuperHyper table?": Value Change {
        n4926 = event-data() -> ()  [unwired: 1 in, 6 out]
        n4927 = stacked-sequence {
          frame #0 {
            n4928 = property on="SuperHyper Steps" class="Tbl (strict)"("Active Cell"=cluster{"Row":i32, "Column":i32} {"Row"=-2, "Column"=-2}, "Cell BG Color"=u32 16448250 ("Active Cell:Cell Background Color")) -> ()  [unwired: 2 in, 2 out]
          }
          frame #1 {
            n4929 = property on="to" class="DigNum (strict)"() -> ("Value"=w6279:dbl)  [unwired: 2 in, 2 out]
            n4930 = property on="from" class="DigNum (strict)"() -> ("Value"=w6280:dbl)  [unwired: 2 in, 2 out]
            n4931 = property on="step" class="DigNum (strict)"() -> ("Value"=w6278:dbl)  [unwired: 2 in, 2 out]
            n4932 = Subtract(x=w6280, y=w6279) -> (x-y=w6286:dbl)
            n4933 = Divide(x=w6286, y=w6278) -> (x/y=w6285:dbl)
            n4934 = Sign(1:w6286) -> (0:w6289:dbl)
            n4935 = Absolute Value(x=w6285) -> (abs(x)=w6284:dbl)
            n4936 = Negate(x=w6289) -> (-x=w6281:dbl)
            n4937 = Round Toward -Infinity(1:w6284) -> (0:w6283:dbl)
            n4938 = Increment(x=w6283) -> (x+1=w6282:dbl)
            n4939 = for {
              N: w6282 -> [_]
              tunnel: w6280 -> [w6295]
              tunnel: w6281 -> [w6296]
              tunnel: w6278 -> [w6298]
              tunnel: [w6292] -> w6287 mode=indexing
              i -> [w6290]
              n4940 = Multiply(x=w6298, y=w6290) -> (x*y=w6297:dbl)
              n4941 = Multiply(x=w6296, y=w6297) -> (x*y=w6294:dbl)
              n4942 = Add(x=w6295, y=w6294) -> (x+y=w6293:dbl)
              n4943 = Number To Fractional String(number=w6293, precision (6)=i16 6) -> (F-format string=w6292:string)  [unwired: 2 in]
            }
            n4944 = Build Array(w6287) -> (w6288:string[][])
            n4945 = Transpose 2D Array(2D array=w6288) -> (transposed array=w6277:string[][])
            n4946 = property on="SuperHyper Steps" class="Tbl (strict)"("Value"=w6277) -> ()  [unwired: 2 in, 2 out]
          }
          frame #2 {
            n4947 = property on="upper limit" class="DigNum (strict)"() -> ("Value"=w6338:dbl)  [unwired: 2 in, 2 out]
            n4948 = property on="lower limit" class="DigNum (strict)"() -> ("Value"=w6339:dbl)  [unwired: 2 in, 2 out]
            n4949 = Subtract(x=w6339, y=w6338) -> (x-y=w6337:dbl)
            n4950 = property on="Down Rate" class="DigNum (strict)"() -> ("Value"=w6334:dbl)  [unwired: 2 in, 2 out]
            n4951 = property on="Up Rate" class="DigNum (strict)"() -> ("Value"=w6336:dbl)  [unwired: 2 in, 2 out]
            n4952 = Absolute Value(x=w6337) -> (abs(x)=w6335:dbl)
            n4953 = property on="step" class="RadioBtnsControl (strict)"() -> ("Value"=w6315:T5)  [unwired: 2 in, 2 out]
            n4954 = Divide(x=w6335, y=w6336) -> (x/y=w6333:dbl)
            n4955 = Divide(x=w6335, y=w6334) -> (x/y=w6332:dbl)
            n4956 = case shown="\"iPS_step\"" w6315 {
              tunnel: [w6340 0.0] -> w6314
              frame "iPS_step" {
                n4957 = property on="step" class="DigNum (strict)"() -> ("Value"=w6344:dbl)  [unwired: 2 in, 2 out]
                n4958 = property on="FieldRate(T/min)" class="DigNum (strict)"() -> ("Value"=w6343:dbl)  [unwired: 2 in, 2 out]
                n4959 = Divide(x=w6344, y=w6343) -> (x/y=w6342:dbl)
                n4960 = Multiply(x=w6342, y=60.0) -> (x*y=w6340:dbl)
              }
              frame "V2400_1_Step".."iTC_step", Default {
              }
            }
            n4961 = property on="Wait Between Step(s)" class="DigNum (strict)"() -> ("Value"=w6329:i32)  [unwired: 2 in, 2 out]
            n4962 = Add(x=w6333, y=w6332) -> (x+y=w6331:dbl)
            n4963 = Multiply(x=w6331, y=60.0) -> (x*y=w6330:dbl)
            n4964 = property on="SuperHyper Steps" class="Tbl (strict)"() -> ("Value"=w6306:string[][])  [unwired: 2 in, 2 out]
            n4965 = property on="HyperLoop Steps" class="Tbl (strict)"() -> ("Value"=w6310:string[][])  [unwired: 2 in, 2 out]
            n4966 = property on="wait between sweeps(s)" class="DigNum (strict)"() -> ("Value"=w6327:u32)  [unwired: 2 in, 2 out]
            n4967 = Add(x=w6330, y=w6329) -> (x+y=w6328:dbl)
            n4968 = property on="Step values" class="Tbl (strict)"() -> ("Value"=w6324:string[][])  [unwired: 2 in, 2 out]
            n4969 = Array Size(array=w6310) -> (size(s)=w6312:i32[])
            n4970 = Array Size(array=w6306) -> (size(s)=w6307:i32[])
            n4971 = Array Size(array=w6324) -> (size(s)=w6323:i32[])
            n4972 = Add(x=w6328, y=w6327) -> (x+y=w6317:dbl)
            n4973 = Index Array(array=w6312, index=0) -> (element=w6313:i32)
            n4974 = Index Array(array=w6307, index=0) -> (element=w6305:i32)
            n4975 = Index Array(array=w6323, index=0) -> (element=w6322:i32)
            n4976 = Add(x=w6317, y=w6314) -> (x+y=w6316:dbl)
            n4977 = Multiply(x=w6322, y=w6316) -> (x*y=w6309:dbl)
            n4978 = Multiply(x=w6313, y=w6309) -> (x*y=w6304:dbl)
            n4979 = Multiply(x=w6305, y=w6304) -> (x*y=w6303:dbl)
            n4980 = Get Date/Time In Seconds() -> (seconds since 1Jan1904=w6326:timestamp)
            n4981 = Add(x=w6303, y=w6326) -> (x+y=w6302:timestamp)
            n4982 = Quotient & Remainder(x=w6303, y=3600.0) -> (x-y*floor(x/y)=w6325:dbl, floor(x/y)=w6301:dbl)
            n4983 = Quotient & Remainder(x=w6325, y=60.0) -> (x-y*floor(x/y)=w6299:dbl, floor(x/y)=w6300:dbl)
            n4984 = property on="HH:" class="DigNum (strict)"("Value"=w6301) -> ()  [unwired: 2 in, 2 out]
            n4985 = property on="Finish Time Super" class="AbsTime (strict)"("Value"=w6302) -> ()  [unwired: 2 in, 2 out]
            n4986 = property on="MM:" class="DigNum (strict)"("Value"=w6300) -> ()  [unwired: 2 in, 2 out]
            n4987 = property on="SS:" class="DigNum (strict)"("Value"=w6299) -> ()  [unwired: 2 in, 2 out]
          }
        }
      }
      event "EstimateTime Hyper": Value Change {
        n4988 = event-data() -> ()  [unwired: 1 in, 6 out]
        n4989 = property on="upper limit" class="DigNum (strict)"() -> ("Value"=w6380:dbl)  [unwired: 2 in, 2 out]
        n4990 = property on="lower limit" class="DigNum (strict)"() -> ("Value"=w6381:dbl)  [unwired: 2 in, 2 out]
        n4991 = Subtract(x=w6381, y=w6380) -> (x-y=w6379:dbl)
        n4992 = property on="Down Rate" class="DigNum (strict)"() -> ("Value"=w6376:dbl)  [unwired: 2 in, 2 out]
        n4993 = property on="Up Rate" class="DigNum (strict)"() -> ("Value"=w6378:dbl)  [unwired: 2 in, 2 out]
        n4994 = Absolute Value(x=w6379) -> (abs(x)=w6377:dbl)
        n4995 = property on="step" class="RadioBtnsControl (strict)"() -> ("Value"=w6357:T5)  [unwired: 2 in, 2 out]
        n4996 = Divide(x=w6377, y=w6378) -> (x/y=w6375:dbl)
        n4997 = Divide(x=w6377, y=w6376) -> (x/y=w6374:dbl)
        n4998 = case shown="\"iPS_step\"" w6357 {
          tunnel: [w6382 0.0] -> w6356
          frame "iPS_step" {
            n4999 = property on="step" class="DigNum (strict)"() -> ("Value"=w6386:dbl)  [unwired: 2 in, 2 out]
